vi "Connect Bool.vi"(8 "Error In":errorcluster, 10 "Signal":string, 11 "Sender In":refnum<class "QObject.lvclass">) -> (0 "Error Out":errorcluster, 2 "Bool Signal":refnum<user-event>, 3 "Sender Out":refnum<class "QObject.lvclass">)   [LabVIEW 2013, in "Template.lvlib" / "LQWidgetEngine.lvclass"]
uses:
  LQWidgetEngine.lvclass
  QObject/QObject.lvclass
  QObject/QObject.lvclass/QObject.ctl
  Connection Action.ctl
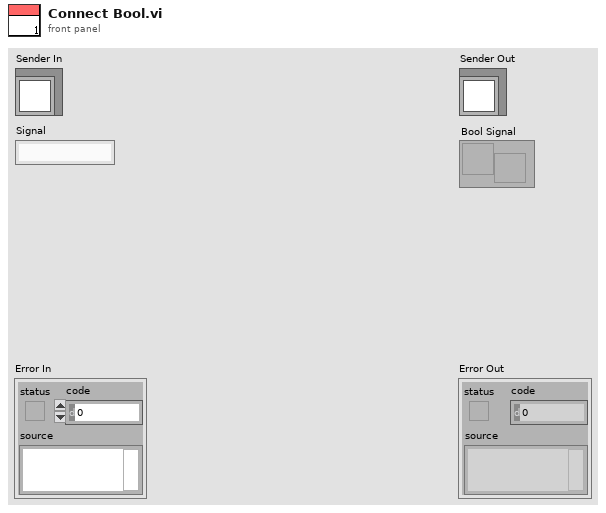
[diagram p1: front panel]
types:
  T1 = typedef "Template.lvlib/LQWidgetEngine.lvclass/Connection Action.ctl" = enum16{"Init", "Add Connection", "Get Connections", "Clean Up"}
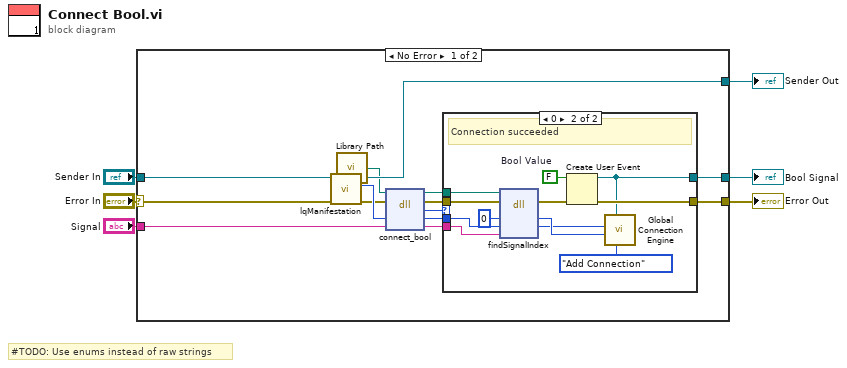
[diagram p0: block diagram]
diagram:
  # "#TODO: Use enums instead of raw strings"
  n1 = case shown="No Error" "Error In" {
    selector: "Error In" -> [w17 w35]
    tunnel: [w13 w35] -> w5
    tunnel: [w19 w34] -> w3
    tunnel: "Sender In" -> [w20 w34]
    tunnel: "Signal" -> [w15 _]
    tunnel: [w12 _] -> w1
    frame No Error {
      n2 = call "lqManifestation.vi"("error in (no error)"=w17, "QObject in"=w20) -> ("error out"=w16:errorcluster, "Manifestation"=w18:u32, "QObject out"=w19:refnum<class "QObject.lvclass">)  [unwired: 7 in]
      n3 = call "Library Path.vi"() -> ("Library Path"=w7:path)
      n4 = dll-call lib="?" fn="connect_bool"(path in=w7, error in=w16, "obj"=w18, "encodedSignal"=w15) -> (path out=w10:path, error out=w14:errorcluster, "errorCode"=w11:i32, "obj"=w9:u32, "encodedSignal"=w8:string)  [unwired: 1 in]
      n5 = case shown="0" w11 {
        tunnel: w14 -> [w21 w31]
        tunnel: [w21 w33] -> w13
        tunnel: [_ w23] -> w12
        tunnel: w10 -> [_ w29]
        tunnel: w9 -> [_ w28]
        tunnel: w8 -> [_ w27]
        frame Default {
          # "#TODO: Create error cluster"
          # "Connection failed"
        }
        frame 0 {
          w32 = FALSE  # Bool Value
          # "Connection succeeded"
          n6 = dll-call lib="?" fn="findSignalIndex"(path in=w29, error in=w31, "retVal"=i64 0, "obj"=w28, "encodedSignal"=w27) -> (error out=w30:errorcluster, "retVal"=w25:i64, "obj"=w24:u32)  [unwired: 3 in, 1 out]
          n7 = Create User Event(user event datatype=w32, error in=w30) -> (user event=w23:refnum<user-event>, error out=w33:errorcluster)
          n8 = call "Global Connection Engine.vi"("Connection Action"=Connection_Action."Add Connection", "Signal Channel"=w23, "Signal Index"=w25, "QObject Refnum"=w24) -> ()  [unwired: 7 in, 1 out]
        }
      }
    }
    frame Error {
    }
  }
  "Error Out" <- w5
  "Sender Out" <- w3
  "Bool Signal" <- w1
